vi "test2.vi"() -> ()   [LabVIEW 2016]
panel:
  out "数组":i32[](array[numeric])
  in  "data":string[][](array[string])=array500x13[6500 elements]
  out "当前要发送的海流计参数":string[][](array[string])
  out "数值":i32
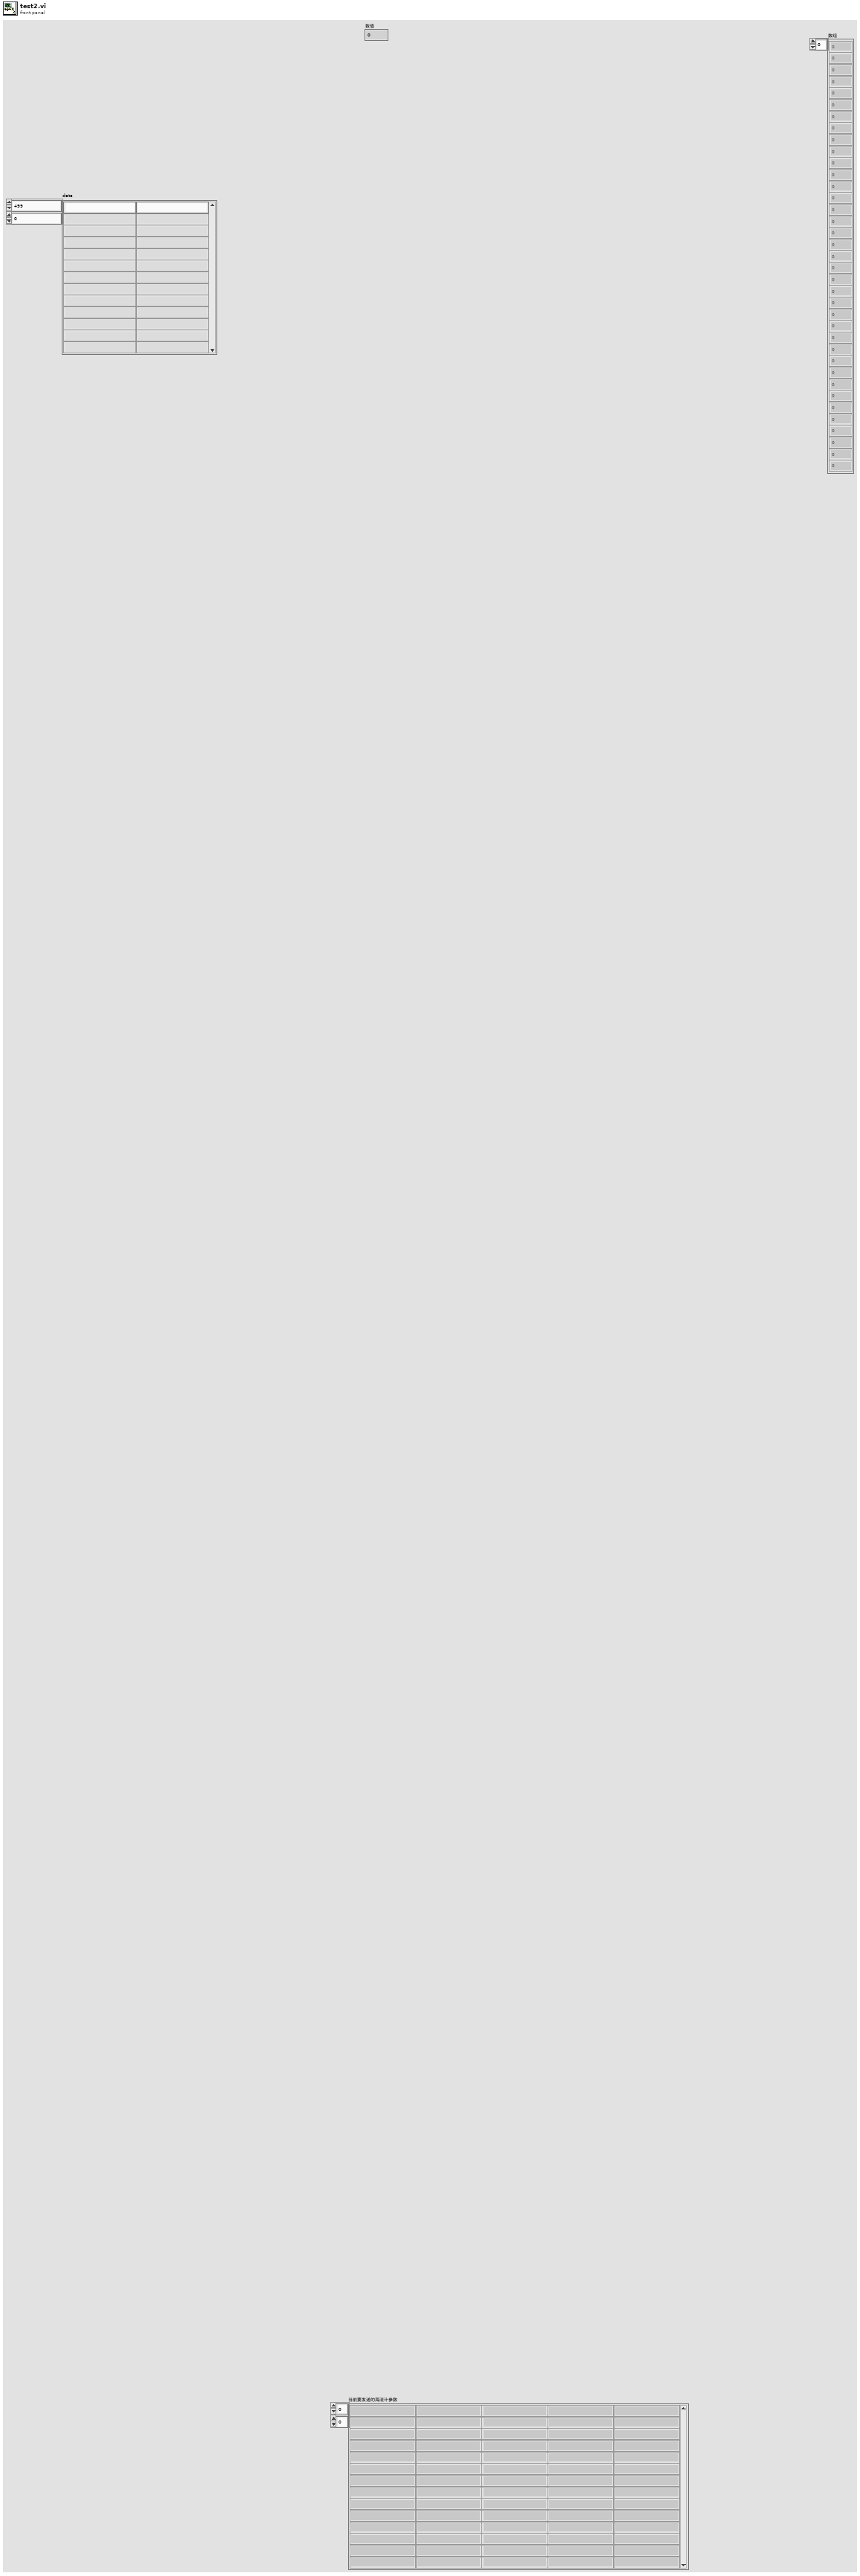
[diagram p1: front panel]
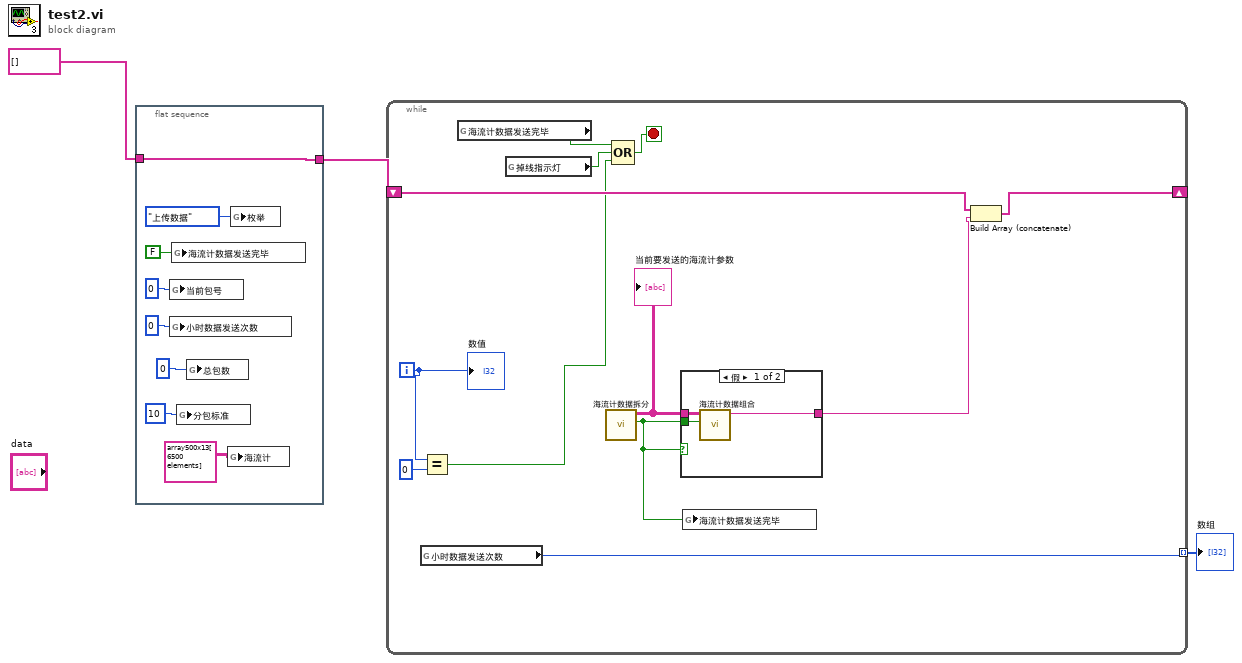
[diagram p0: block diagram]
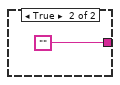
[diagram p2: hidden frame]
diagram:
  n1 = flat-sequence {
    tunnel: [w7] -> w2
    tunnel: string[] [] -> [w7]
    frame #0 {
      n2 = global write "全局 数据数组大小.vi" "当前包号"(0 ("当前包号")) -> ()
      n3 = global write "全局 小时数据发送次数.vi" "小时数据发送次数"(0 ("小时数据发送次数")) -> ()
      n4 = global write "全局 数据数组大小.vi" "海流计数据发送完毕"(FALSE ("海流计数据发送完毕")) -> ()
      n5 = global write "全局 数据数组大小.vi" "分包标准"(10 ("当前包号")) -> ()
      n6 = global write "全局 数据数组大小.vi" "总包数"(0 ("当前包号")) -> ()
      n7 = global write "全局 所有参数.vi" "海流计"(string[][] array500x13[6500 elements] ("data")) -> ()
      n8 = global write "全局1.vi" "枚举"(enum16{"返回请求应答", "上传数据", "返回执行结果"}."上传数据" ("枚举")) -> ()
    }
  }
  n9 = while {
    shift-right: [w19] -> _
    shift-left: w2 -> [w20]
    tunnel: [w13] -> w1 mode=indexing
    i -> [w15]
    stop <- w22 stop-if-true
    n10 = global read "全局 小时数据发送次数.vi" "小时数据发送次数"() -> (w13:i32)
    n11 = Equal?(x=w15, y=0) -> (x = y?=w12:bool)
    n12 = global read "全局 数据数组大小.vi" "海流计数据发送完毕"() -> (w21:bool)
    n13 = global read "全局 数据发送重叠.vi" "掉线指示灯"() -> (w23:bool)
    n14 = call "海流计数据拆分.vi"() -> ("不再发送"=w17:bool, "当前要发送的海流计参数"=w18:string[][])  [unwired: 10 in]
    "当前要发送的海流计参数" <- w18
    n15 = Compound Arithmetic op=OR ("复合运算")(w21, w23, w12) -> (w22:bool)
    n16 = case shown="假" w17 {
      tunnel: [w26 ""] -> w16
      tunnel: w18 -> [w25 _]
      tunnel: w17 -> [w24 _]
      frame False {
        n17 = call "海流计数据组合.vi"("不再发送"=w24, "要发送的海流计参数"=w25) -> ("发送的信息"=w26:string)  [unwired: 9 in]
      }
      frame True {
      }
    }
    n18 = global write "全局 数据数组大小.vi" "海流计数据发送完毕"(w17) -> ()
    n19 = Build Array (concatenate)(w20, w16) -> (w19:string[])
    "数值" <- w15
  }
  "数组" <- w1
